vi "fgt set pressure Unit.vi"(8 "error in (no error)":errorcluster, 10 "unit":T1, 11 "presureIndex":u32) -> (0 "error out":errorcluster)   [LabVIEW 2016, in "fgt_SDK.lvlib"]
doc: "Set pressure unit on selected pressure device, default value is \"mbar\". If type is invalid an error is returned.\nEvery pressure read value and sent command will then use this unit.\nExample of type: \"mbar\", \"millibar\", \"kPa\" ..."
uses:
  fgt_SDK.lvlib
  TypeDefs/fgt_PRESSURE_UNIT.ctl
  dlls/fgt_SDK_32.dll
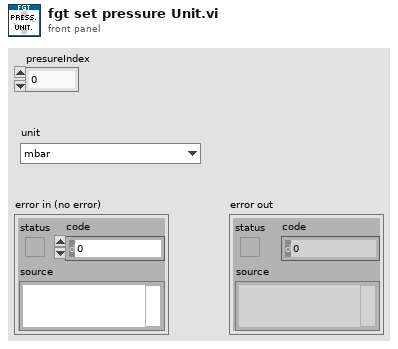
[diagram p1: front panel]
types:
  T1 = typedef "fgt_SDK.lvlib/fgt_PRESSURE_UNIT.ctl" = enum16{"mbar", "kPa", "PSI"}
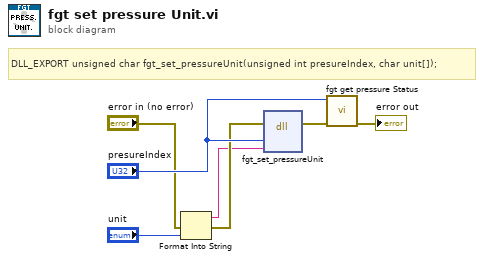
[diagram p0: block diagram]
diagram:
  # "DLL_EXPORT unsigned char fgt_set_pressureUnit(unsigned int presureIndex, char unit[]);"
  n1 = Format Into String(error in="error in (no error)", "unit") -> (resulting string=w1:string, error out=w2:errorcluster)  [unwired: 2 in]
  n2 = dll-call lib="PTH2Zabs D\nMes DocumentsDéveloppementFluigentSDKsfgt-sdk-labviewdllsfgt_SDK_*.*" fn="fgt_set_pressureUnit"(error in=w2, "presureIndex"="presureIndex", "unit"=w1) -> (error out=w7:errorcluster)  [unwired: 5 in, 1 out]
  n3 = call "fgt get pressure Status.vi"("error in (no error)"=w7, "pressureIndex"="presureIndex") -> ("error out"=→"error out":errorcluster)  [unwired: 9 in]
